vi "MVP Valve Operate.vi"(0 "VISA resource name":refnum<visa-resource-name>="VALVE", 7 "Valve # (1=a, 2=b, ....  0 = no prefix)":u8=1, 9 "Valve position in":u8=2, 11 "error in (no error)":errorcluster) -> (4 "VISA resource name out":refnum<visa-resource-name>, 10 "Valve position out":u8, 15 "error out":errorcluster)   [LabVIEW 2015]
doc: "Reads a response from the pump affter a command is sent\n\nModified from original which is Copyright 2005, National Instruments Corporation"
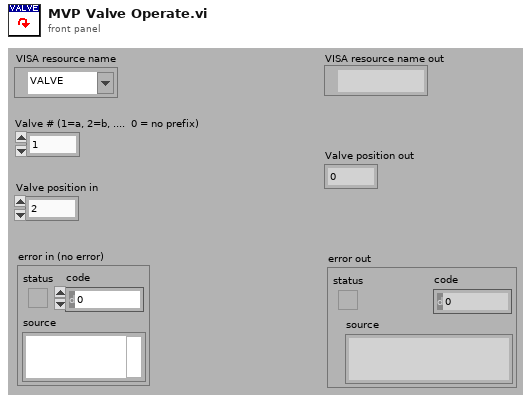
[diagram p1: front panel]
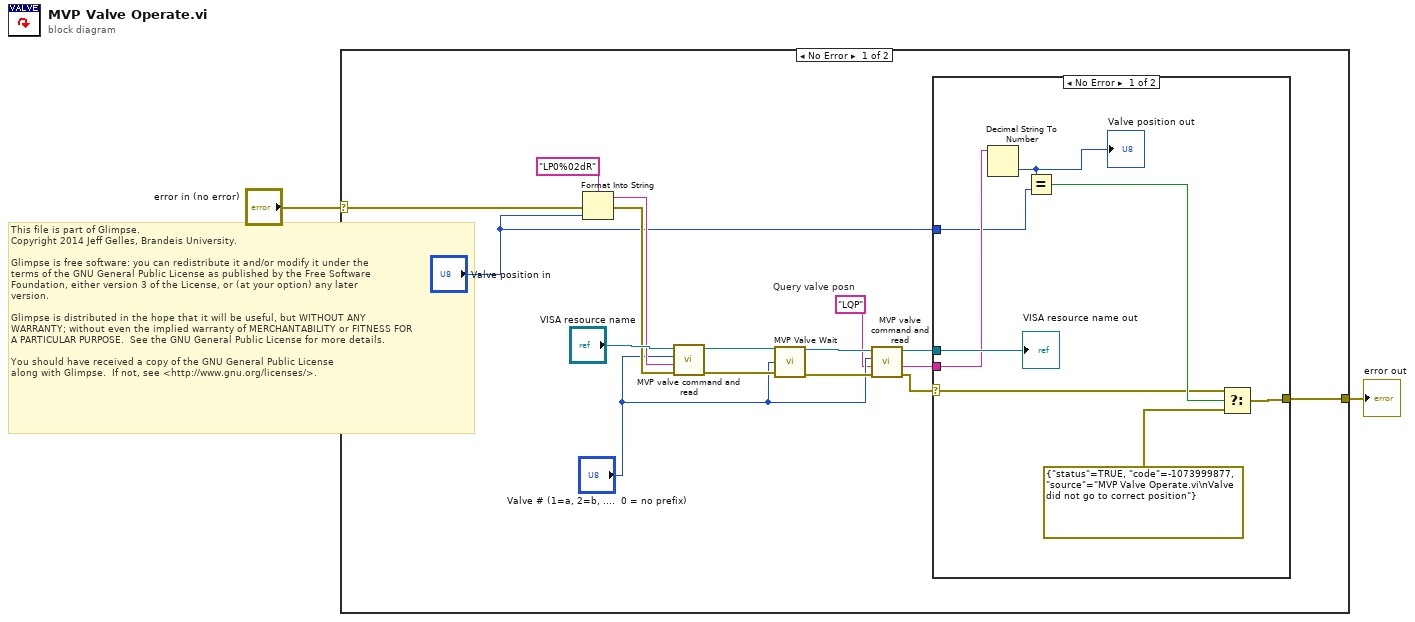
[diagram p0: block diagram]
diagram:
  # "This file is part of Glimpse. \nCopyright 2014 Jeff Gelles, Brandeis University.    \n\nGlimpse is free software: you can redistribute it and/or modify it under the \nterms of the GNU General Public License as published by the Free Software \nFoundation, either version 3 of the License, or (at your option) any later \nversion.\n\nGlimpse is distributed in the hope that it will be useful, but WITHOUT ANY \nWARRANTY; without even the implied warranty of MERCHANTABILITY or FITNESS FOR \nA PARTICULAR PURPOSE.  See the GNU General Public License for more details.\n\nYou should have received a copy of the GNU General Public License\nalong with Glimpse.  If not, see <http://www.gnu.org/licenses/>."
  n1 = case shown="No Error" "error in (no error)" {
    selector: "error in (no error)" -> [w4 w28]
    tunnel: [w17 w28] -> w2
    frame No Error {
      w7 = "LQP"  # Query valve posn
      n2 = Format Into String(format string="LP0%02dR", error in=w4, "Valve position in") -> (resulting string=w15:string, error out=w14:errorcluster)  [unwired: 1 in]
      n3 = call "MVP valve command and read.vi"("error in"=w14, "command\n(w/o pump # prefix)"=w15, "Valve # (1=a, 2=b, ....  0 = no prefix)"="Valve # (1=a, 2=b, ....  0 = no prefix)", "VISA resource name"="VISA resource name") -> ("error out"=w11:errorcluster, "VISA resource name out"=w13:refnum<visa-resource-name>)  [unwired: 3 out]
      n4 = call "MVP Valve Wait.vi"("VISA resource name"=w13, "Valve # (1=a, 2=b, ....  0 = no prefix)"="Valve # (1=a, 2=b, ....  0 = no prefix)", "error in (no error)"=w11) -> ("VISA resource name out"=w12:refnum<visa-resource-name>, "error out"=w10:errorcluster)  [unwired: 11 out]
      n5 = call "MVP valve command and read.vi"("error in"=w10, "command\n(w/o pump # prefix)"=w7, "Valve # (1=a, 2=b, ....  0 = no prefix)"="Valve # (1=a, 2=b, ....  0 = no prefix)", "VISA resource name"=w12) -> ("error out"=w3:errorcluster, "Output String"=w6:string, "VISA resource name out"=w9:refnum<visa-resource-name>)  [unwired: 2 out]
      n6 = case shown="No Error" w3 {
        selector: w3 -> [w19 w27]
        tunnel: [w26 w27] -> w17
        tunnel: w9 -> [w25 _]
        tunnel: w6 -> [w24 _]
        tunnel: "Valve position in" -> [w22 _]
        frame No Error {
          n7 = Decimal String To Number(string=w24) -> (number=w23:i32)  [unwired: 3 out]
          "Valve position out" <- w23
          n8 = Equal?(x=w23, y=w22) -> (x = y?=w20:bool)
          n9 = Select(t=w19, s=w20, f=errorcluster {"status"=TRUE, "code"=-1073999877, "source"="MVP Valve Operate.vi\nValve did not go to correct position"} ("t")) -> (s? t:f=w26:errorcluster)
          "VISA resource name out" <- w25
        }
        frame Error {
        }
      }
    }
    frame Error {
    }
  }
  "error out" <- w2
